vi "Split Path Tokens.vi"(11 "Path":string) -> (3 "Tokens":string[](array[string]))   [LabVIEW 2020, in "PathTree.lvlib" / "PathTreeNode.lvclass"]
uses:
  PathTreeNode.lvclass
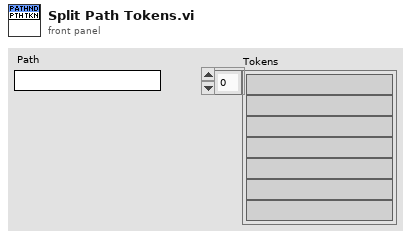
[diagram p1: front panel]
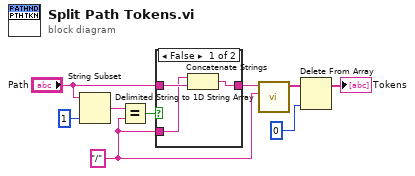
[diagram p0: block diagram]
diagram:
  w5 = "/" ("y")
  n1 = String Subset(string="Path", length (rest)=1 ("length (rest)")) -> (substring=w8:string)  [unwired: 1 in]
  n2 = Equal?(x=w8, y=w5) -> (x = y?=w7:bool)
  n3 = case shown="False" w7 {
    tunnel: "Path" -> [w12 w13]
    tunnel: w5 -> [w11 _]
    tunnel: [w10 w13] -> w6
    frame False {
      n4 = Concatenate Strings(w11, w12) -> (w10:string)
    }
    frame True {
    }
  }
  n5 = call <vilib>:"Delimited String to 1D String Array.vi"("delimiter"=w5, "delimited string"=w6) -> ("string array"=w4:string[])  [unwired: 9 in]
  n6 = Delete From Array(array=w4, index=0) -> (array with subset deleted=→"Tokens":string[])  [unwired: 1 in, 1 out]
